vi "Open HW References.vi"(11 "Module Azimuth Config Data":T1) -> (0 "Error Out":errorcluster, 1 "Error Out":errorcluster, 2 "Module Drive Ref Out":T3, 3 "Module Steer Ref Out":T3)   [LabVIEW 2023, in "Swerve-SteerSRX-DriveSpark-AbsAnalog_ACT.lvlib"]
uses:
  Swerve-SteerSRX-DriveSpark-AbsAnalog_ACT.lvlib
  <vilib>/Rock Robotics/WPI/MotorControl/WPI_MotorControlDeviceRef.ctl
  <vilib>/Rock Robotics/WPI/MotorControl/WPI_MotorControlType.ctl
  <vilib>/Rock Robotics/SystemInterfaces/DIO/FPGA_DIOPWMChannel.ctl
  <vilib>/Rock Robotics/WPI/PWM/WPI_PWMDeadband.ctl
  <vilib>/Rock Robotics/SystemInterfaces/DIO/FPGA_DIOChannel.ctl
  Cluster_Config Specific Data.ctl
  Shared Code/TypeDefs/ENUM_Module Position.ctl
  <vilib>/Rock Robotics/WPI/ThirdParty/REV Robotics/REVLib/Typedef/Spark MAX Motor Type.ctl
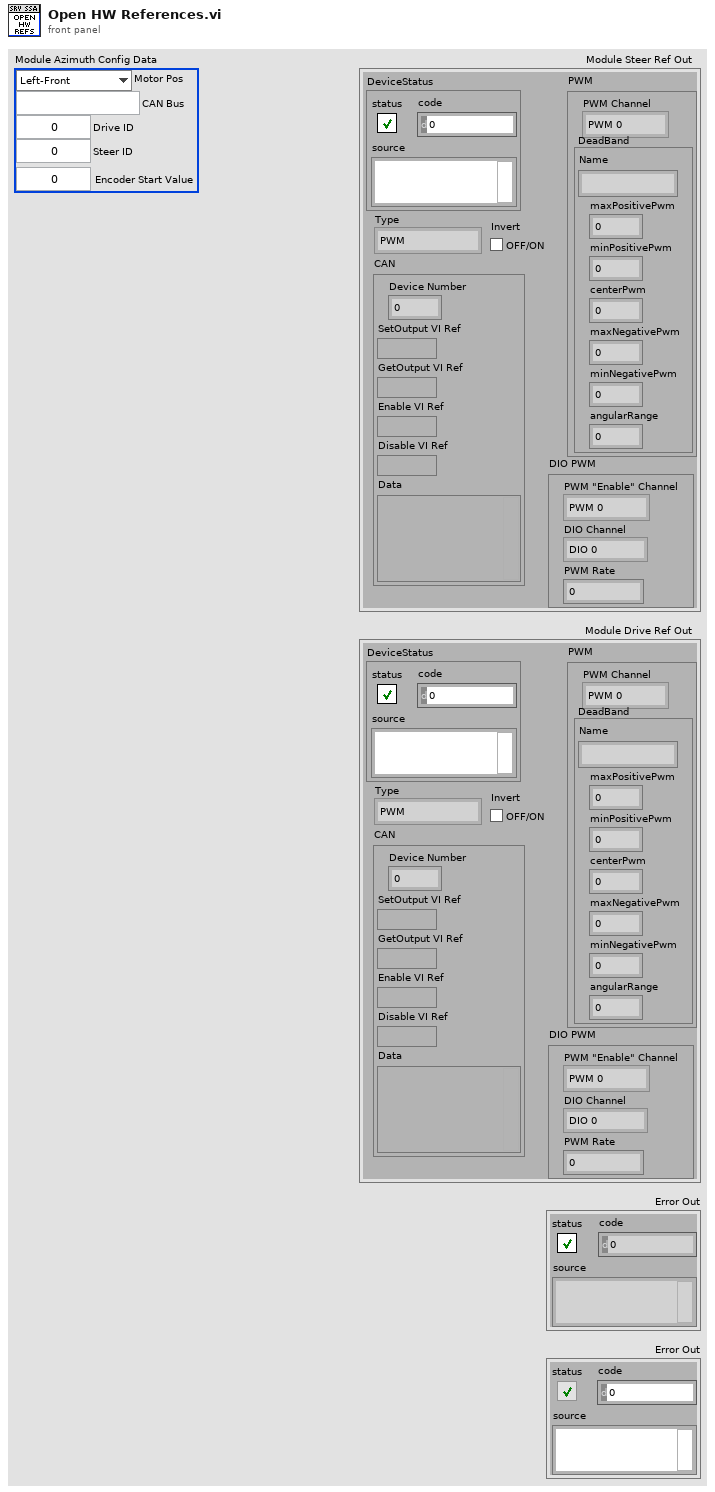
[diagram p1: front panel]
types:
  T1 = typedef "Swerve-SteerSRX-DriveSpark-AbsAnalog_ACT.lvlib/Cluster_Config Specific Data.ctl" = cluster{"Motor Pos":T2, "CAN Bus":string, "Drive ID":u8, "Steer ID":u8, "Encoder Start Value":dbl}
  T2 = typedef "ENUM_Module Position.ctl" = enum16{"Left-Front", "Right-Front", "Left-Back", "Right-Back"}
  T3 = typedef "WPI_MotorControlDeviceRef.ctl" = cluster{"DeviceStatus":errorcluster, "Type":T4, "PWM":cluster{"PWM Channel":T5, "DeadBand":T6}, "CAN":cluster{"Device Number":u8, "SetOutput VI Ref":variant, "GetOutput VI Ref":variant, "Enable VI Ref":variant, "Disable VI Ref":variant, "Data":variant}, "Invert":bool, "DIO PWM":cluster{"PWM \"Enable\" Channel":T5, "DIOChannel":T7, "PWM Rate":dbl}}
  T4 = typedef "WPI_MotorControlType.ctl" = enum16{"PWM", "CAN", "DIO PWM"}
  T5 = typedef "FPGA_DIOPWMChannel.ctl" = enum8{"PWM 0", "PWM 1", "PWM 2", "PWM 3", "PWM 4", "PWM 5", "PWM 6", "PWM 7", "PWM 8", "PWM 9", "PWM MXP 0", "PWM MXP 1", "PWM MXP 2", "PWM MXP 3", "PWM MXP 4", "PWM MXP 5", "PWM MXP 6", "PWM MXP 7", "PWM MXP 8", "PWM MXP 9", "Invalid"}
  T6 = typedef "WPI_PWMDeadband.ctl" = cluster{"Name":string, "maxPositivePwm":i32, "minPositivePwm":i32, "centerPwm":i32, "maxNegativePwm":i32, "minNegativePwm":i32, "angularRange":u16}
  T7 = typedef "FPGA_DIOChannel.ctl" = enum8{"DIO 0", "DIO 1", "DIO 2", "DIO 3", "DIO 4", "DIO 5", "DIO 6", "DIO 7", "DIO 8", "DIO 9", "DIO MXP 0", "DIO MXP 1", "DIO MXP 2", "DIO MXP 3", "DIO MXP 4", "DIO MXP 5", "DIO MXP 6", "DIO MXP 7", "DIO MXP 8", "DIO MXP 9", "DIO MXP 10", "DIO MXP 11", "DIO MXP 12", "DIO MXP 13", "DIO MXP 14", "DIO MXP 15", "SPI Port CS1", "SPI Port CS2", "SPI Port CS3", "SPI Port MISO", "SPI Port MOSI", "Invalid"}
  T8 = typedef "Spark MAX Motor Type.ctl" = enum16{"Brushed", "Brushless"}
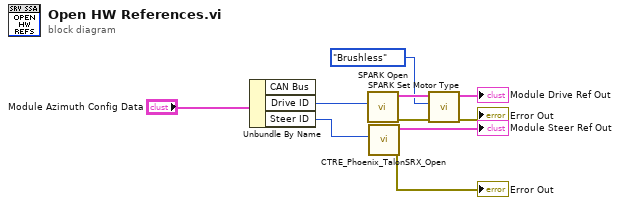
[diagram p0: block diagram]
diagram:
  n1 = Unbundle By Name("Module Azimuth Config Data") -> ("Drive ID"=w8:u8, "Steer ID"=w9:u8)  [unwired: 1 out]
  n2 = call <vilib>:"SPARK Open.vi"("Device Number"=w8) -> ("error out"=w2:errorcluster, "MotorControlDeviceRef"=w4:T3)  [unwired: 9 in]
  n3 = call <vilib>:"CTRE_Phoenix_TalonSRX_Open.vi"("Device Number"=w9) -> ("error out"=→"Error Out":errorcluster, "PhoenixMotorControlDevRef"=→"Module Steer Ref Out":T3)  [unwired: 9 in]
  n4 = call <vilib>:"SPARK Set Motor Type.vi"("error in (no error)"=w2, "Motor Type"=Spark_MAX_Motor_Type."Brushless", "MotorControlDevRef"=w4) -> ("error out"=→"Error Out":errorcluster, "MotorControlDeviceRef"=→"Module Drive Ref Out":T3)  [unwired: 7 in]
